vi "json.update.vi"(8 "error in":errorcluster, 9 "Object Name":string="timestampMetadata", 10 "JSON in":string, 11 "timestampMetadata in":refnum<class "timestampMetadata.lvclass">) -> (0 "error out":errorcluster, 2 "JSON out":string, 3 "timestampMetadata out":refnum<class "timestampMetadata.lvclass">)   [LabVIEW 2020, in "timestampMetadata.lvclass"]
uses:
  timestampMetadata.lvclass
  <vilib>/JDP Science/JSONtext/Get all Object Items.vi
  <vilib>/JDP Science/JSONtext/Set Multiple Object Items.vi
  <vilib>/JDP Science/JSONtext/JSONtext.lvlib
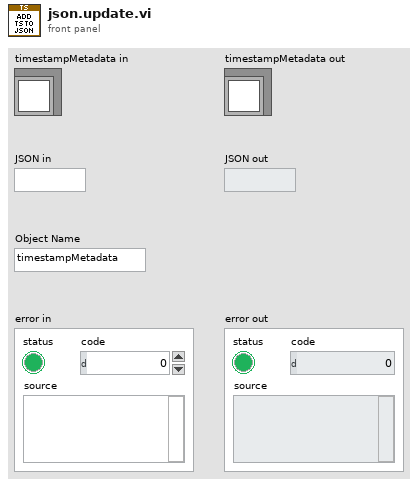
[diagram p1: front panel]
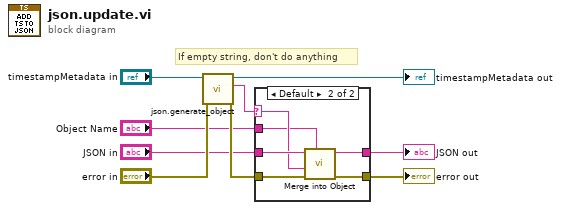
[diagram p0: block diagram]
diagram:
  # "If empty string, don't do anything"
  n1 = call-dynamic "json.generate_object.vi"("error in"="error in", "timestampMetadata in"="timestampMetadata in") -> ("error out"=w6:errorcluster, "JSON Object"=w7:string, "timestampMetadata out"=→"timestampMetadata out":refnum<class "timestampMetadata.lvclass">)  [unwired: 7 in]
  n2 = case shown="Default" w7 {
    selector: w7 -> [_ w16]
    tunnel: "JSON in" -> [w11 w17]
    tunnel: w6 -> [w10 w15]
    tunnel: [w11 w14] -> w5
    tunnel: "Object Name" -> [_ w13]
    tunnel: [w10 w12] -> w4
    frame "" {
    }
    frame Default {
      n3 = call <vilib>:"Merge into Object.vi"("$Path or Item Name"=w13, "error in (no error)"=w15, "JSON Object to Merge"=w16, "JSON"=w17) -> ("error out"=w12:errorcluster, "<JSON>"=w14:string)  [unwired: 5 in]
    }
  }
  "error out" <- w4
  "JSON out" <- w5
